vi "Read Method Information.vi"(8 "error in (no error)":errorcluster, 9 "Method":string, 10 "Name":string, 11 "TwinCAT ADS in":refnum<class "TwinCAT ADS.lvclass">) -> (0 "error out":errorcluster, 1 "Method Information":T1 {"Parameters"."Parameter Flags" items=["In"=1, "Out"=2, "ByReference"=4, "MaskIn"=5, "MaskOut"=6]}, 3 "TwinCAT ADS out":refnum<class "TwinCAT ADS.lvclass">)   [LabVIEW 2018, in "TwinCAT ADS.lvclass"]
uses:
  TwinCAT ADS.lvclass
  Controls/Method Information.ctl
  Controls/Method Parameter Information.ctl
  TwinCAT.Ads
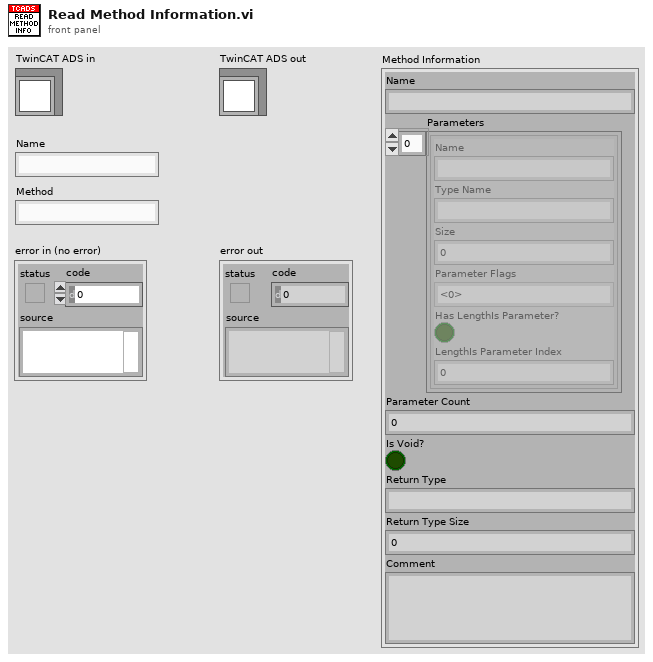
[diagram p1: front panel]
types:
  T1 = typedef "TwinCAT ADS.lvclass/Method Information.ctl" = cluster{"Name":string, "Parameters":T2[], "Parameter Count":i32, "Is Void?":bool, "Return Type":string, "Return Type Size":i32, "Comment":string}
  T2 = typedef "TwinCAT ADS.lvclass/Method Parameter Information.ctl" = cluster{"Name":string, "Type Name":string, "Size":i32, "Parameter Flags":u32, "Has LengthIs Parameter?":bool, "LengthIs Parameter Index":i32}
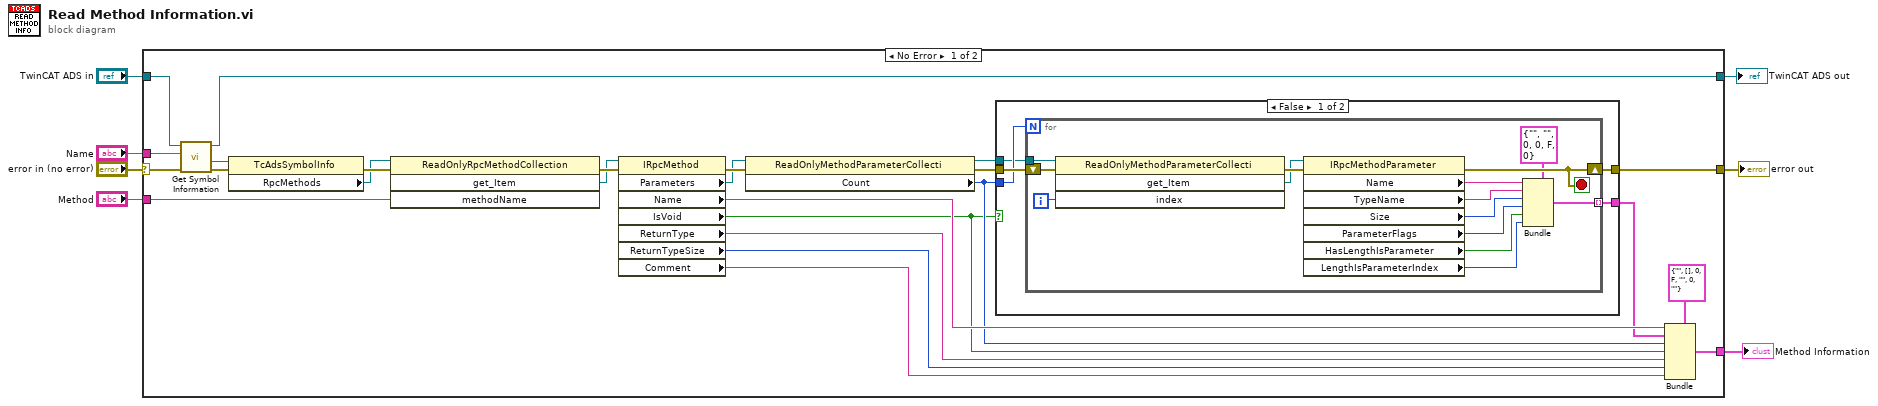
[diagram p0: block diagram]
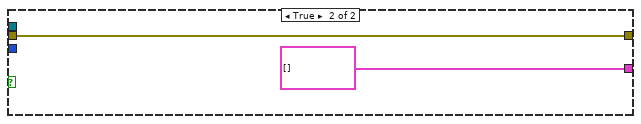
[diagram p2: hidden frame]
diagram:
  n1 = case shown="No Error" "error in (no error)" {
    selector: "error in (no error)" -> [w30 w55]
    tunnel: [w16 w55] -> w6
    tunnel: [w14 w54] -> w4
    tunnel: "TwinCAT ADS in" -> [w8 w54]
    tunnel: "Name" -> [w31 _]
    tunnel: "Method" -> [w25 _]
    tunnel: [w15 _] -> w1
    frame No Error {
      n2 = call-dynamic "Get Symbol Information.vi"("error in (no error)"=w30, "Name"=w31, "TwinCAT ADS in"=w8) -> ("error out"=w29:errorcluster, "Symbol Info"=w28:refnum<k24>, "TwinCAT ADS out"=w14:refnum<class "TwinCAT ADS.lvclass">)  [unwired: 6 in]
      n3 = property class="TcAdsSymbolInfo"(reference=w28, error in=w29) -> (error out=w27:errorcluster, "RpcMethods"=w26:refnum<k24>)  [unwired: 1 out]
      n4 = invoke class="ReadOnlyRpcMethodCollection" method="get_Item"(reference=w26, error in=w27, "methodName"=w25) -> (error out=w24:errorcluster, "get_Item"=w23:refnum<k24>)  [unwired: 1 in, 2 out]
      n5 = property class="IRpcMethod"(reference=w23, error in=w24) -> (error out=w22:errorcluster, "Parameters"=w21:refnum<k24>, "Name"=w19:string, "IsVoid"=w12:bool, "ReturnType"=w11:string, "ReturnTypeSize"=w10:i32, "Comment"=w9:string)  [unwired: 1 out]
      n6 = property class="ReadOnlyMethodParameterCollecti"(reference=w21, error in=w22) -> (reference out=w20:refnum<k24>, error out=w32:errorcluster, "Count"=w13:i32)
      n7 = case shown="False" w12 {
        tunnel: w32 -> [w37 w52]
        tunnel: w13 -> [w36 _]
        tunnel: w20 -> [w35 _]
        tunnel: [w34 T2[] []] -> w18
        tunnel: [w33 w52] -> w16
        frame False {
          n8 = for {
            N: w36 -> [_]
            tunnel: w35 -> [w50]
            shift-right: [w39] -> w33
            shift-left: w37 -> [w51]
            tunnel: [w40] -> w34 mode=indexing
            i -> [w49]
            stop <- w39 stop-if-true
            n9 = invoke class="ReadOnlyMethodParameterCollecti" method="get_Item"(reference=w50, error in=w51, "index"=w49) -> (error out=w48:errorcluster, "get_Item"=w47:refnum<k24>)  [unwired: 1 in, 2 out]
            n10 = property class="IRpcMethodParameter"(reference=w47, error in=w48) -> (error out=w39:errorcluster, "Name"=w46:string, "TypeName"=w45:string, "Size"=w44:i32, "ParameterFlags"=w41:u32, "HasLengthIsParameter"=w43:bool, "LengthIsParameterIndex"=w42:i32)  [unwired: 1 out]
            n11 = Bundle(cluster=T2 {"Name"="", "Type Name"="", "Size"=0, "Parameter Flags"=0, "Has LengthIs Parameter?"=FALSE, "LengthIs Parameter Index"=0} ("Method Parameter Infomation"), "Name"=w46, "Type Name"=w45, "Size"=w44, "Parameter Flags"=w41, "Has LengthIs Parameter?"=w43, "LengthIs Parameter Index"=w42) -> (w40:T2)
          }
        }
        frame True {
        }
      }
      n12 = Bundle(cluster=T1 {"Name"="", "Parameters"=[], "Parameter Count"=0, "Is Void?"=FALSE, "Return Type"="", "Return Type Size"=0, "Comment"=""} ("Method Information"), "Name"=w19, "Parameters"=w18, "Parameter Count"=w13, "Is Void?"=w12, "Return Type"=w11, "Return Type Size"=w10, "Comment"=w9) -> (w15:T1)
    }
    frame Error {
    }
  }
  "error out" <- w6
  "TwinCAT ADS out" <- w4
  "Method Information" <- w1
